vi "Set Time Limit.vi"() -> (0 "Time Limit":dbl)   [LabVIEW 2014]
panel:
  in  "Cancel Button":bool
  in  "OK Button":bool
  in  "Numeric":i32 min=0
  # "Please enter the time limit of Simulation."
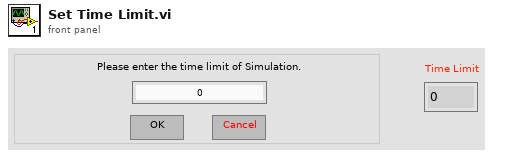
[diagram p1: front panel]
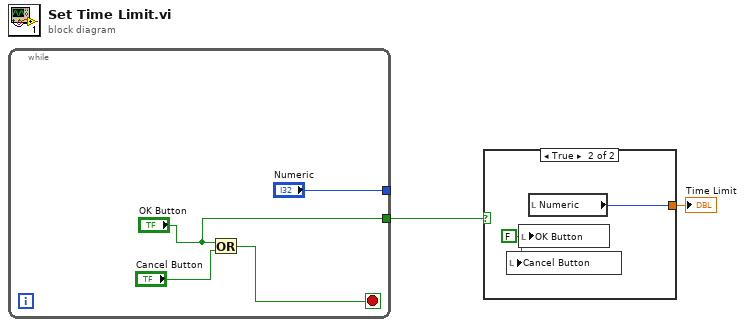
[diagram p0: block diagram]
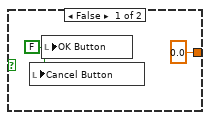
[diagram p2: hidden frame]
diagram:
  n1 = while {
    tunnel: ["Numeric"] -> _
    tunnel: ["OK Button"] -> w2
    stop <- w4 stop-if-true
    n2 = Or(x="OK Button", y="Cancel Button") -> (x .or. y?=w4:bool)
  }
  n3 = case shown="True" w2 {
    tunnel: [0.0 ("Numeric") w9] -> w1
    frame False {
      w7 = FALSE ("OK Button")
      n4 = local write "Cancel Button"(w7) -> ()
      n5 = local write "OK Button"(w7) -> ()
    }
    frame True {
      w10 = FALSE ("OK Button")
      n6 = local write "Cancel Button"(w10) -> ()
      n7 = local write "OK Button"(w10) -> ()
      n8 = local read "Numeric"() -> (w9:i32)
    }
  }
  "Time Limit" <- w1
